vi "Find Local NHMFL ENET Address.vi"(8 "error in (no error)":errorcluster) -> (0 "error out":errorcluster, 3 "Ethernet Address":u32 format="%.0x")   [LabVIEW 2023]
doc: "Author: Scott Hannahs <sth@magnet.fsu.edu>\nCopyright 2018 Florida State University, All rights reserved."
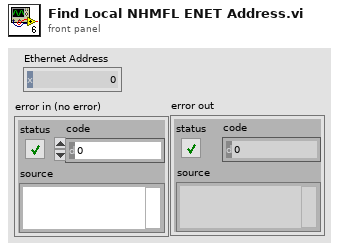
[diagram p1: front panel]
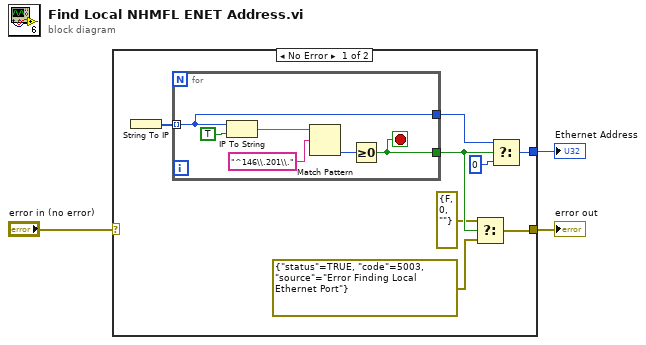
[diagram p0: block diagram]
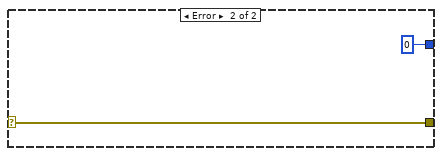
[diagram p2: hidden frame]
diagram:
  n1 = case shown="No Error" "error in (no error)" {
    selector: "error in (no error)" -> [_ w18]
    tunnel: [w10 u32 0 ("f")] -> w3
    tunnel: [w6 w18] -> w1
    frame No Error {
      n2 = String To IP() -> (0:w11:u32[])  [unwired: 1 in]
      n3 = for {
        tunnel: w11 -> [w17] mode=indexing
        tunnel: [w17] -> w9
        tunnel: [w12] -> w7
        stop <- w12 stop-if-true
        n4 = IP To String(1:TRUE ("dot notation? (F)"), 2:w17) -> (0:w15:string)
        n5 = Match Pattern(string=w15, regular expression="^146\\.201\\.") -> (offset past match=w13:i32)  [unwired: 1 in, 3 out]
        n6 = Greater Or Equal To 0?(x=w13) -> (x >= 0?=w12:bool)
      }
      n7 = Select(t=errorcluster {"status"=FALSE, "code"=0, "source"=""} ("error IO"), s=w7, f=errorcluster {"status"=TRUE, "code"=5003, "source"="Error Finding Local Ethernet Port"}) -> (s? t:f=w6:errorcluster)
      n8 = Select(t=w9, s=w7, f=u32 0) -> (s? t:f=w10:u32)
    }
    frame Error {
    }
  }
  "Ethernet Address" <- w3
  "error out" <- w1
